vi "5492_AutonomousTurn.vi"(8 "error in (no error)":errorcluster, 10 "Yaw Goallll":dbl) -> (0 "error out (no error)":errorcluster)   [LabVIEW 2017]
uses:
  Public/Documents/Cross The Road Electronics/Phoenix-LabVIEW/Motor Controller/Controls/CTRE_Phoenix_MotorControl_ControlMode.ctl
  <vilib>/Rock Robotics/WPI/Utilities/WPI_GetSetVariantRefNum.vi
  <vilib>/Rock Robotics/WPI/RobotDrive/WPI_RobotDriveSafetyCheck.vi
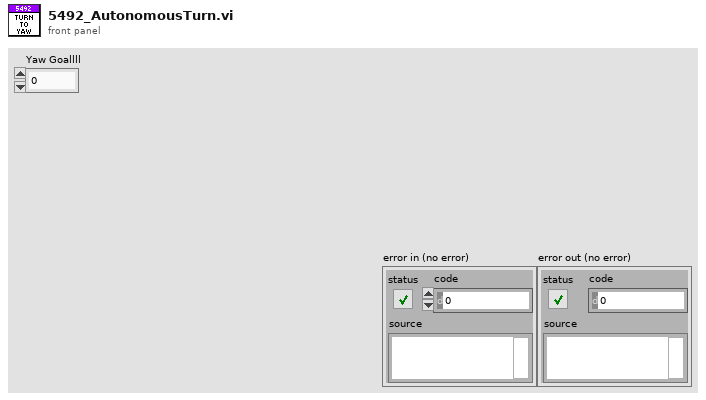
[diagram p1: front panel]
types:
  T1 = typedef "CTRE_Phoenix_MotorControl_ControlMode.ctl" = u16
  T2 = cluster{"Yaw":dbl, "Roll":dbl, "Pitch":dbl, "Heading":dbl, "Fused Heading":dbl}
  T3 = typedef "WPI_RobotDriveDevRef.ctl" = cluster{"DevStatus":errorcluster, "Motors[]":T4[], "Square Inputs":bool, "Max Output":dbl}
  T4 = typedef "WPI_MotorControlDeviceRef.ctl" = cluster{"DeviceStatus":errorcluster, "Type":T5, "PWM":cluster{"PWM Channel":T6, "DeadBand":T7}, "CAN":cluster{"Device Number":u8, "SetOutput VI Ref":variant, "GetOutput VI Ref":variant, "Enable VI Ref":variant, "Disable VI Ref":variant, "Data":variant}, "Invert":bool, "DIO PWM":cluster{"PWM \"Enable\" Channel":T6, "DIOChannel":T8, "PWM Rate":dbl}}
  T5 = typedef "WPI_MotorControlType.ctl" = enum16{"PWM", "CAN", "DIO PWM"}
  T6 = typedef "FPGA_DIOPWMChannel.ctl" = enum8{"PWM 0", "PWM 1", "PWM 2", "PWM 3", "PWM 4", "PWM 5", "PWM 6", "PWM 7", "PWM 8", "PWM 9", "PWM MXP 0", "PWM MXP 1", "PWM MXP 2", "PWM MXP 3", "PWM MXP 4", "PWM MXP 5", "PWM MXP 6", "PWM MXP 7", "PWM MXP 8", "PWM MXP 9", "Invalid"}
  T7 = typedef "WPI_PWMDeadband.ctl" = cluster{"Name":string, "maxPositivePwm":i32, "minPositivePwm":i32, "centerPwm":i32, "maxNegativePwm":i32, "minNegativePwm":i32, "angularRange":u16}
  T8 = typedef "FPGA_DIOChannel.ctl" = enum8{"DIO 0", "DIO 1", "DIO 2", "DIO 3", "DIO 4", "DIO 5", "DIO 6", "DIO 7", "DIO 8", "DIO 9", "DIO MXP 0", "DIO MXP 1", "DIO MXP 2", "DIO MXP 3", "DIO MXP 4", "DIO MXP 5", "DIO MXP 6", "DIO MXP 7", "DIO MXP 8", "DIO MXP 9", "DIO MXP 10", "DIO MXP 11", "DIO MXP 12", "DIO MXP 13", "DIO MXP 14", "DIO MXP 15", "SPI Port CS1", "SPI Port CS2", "SPI Port CS3", "SPI Port MISO", "SPI Port MOSI", "Invalid"}
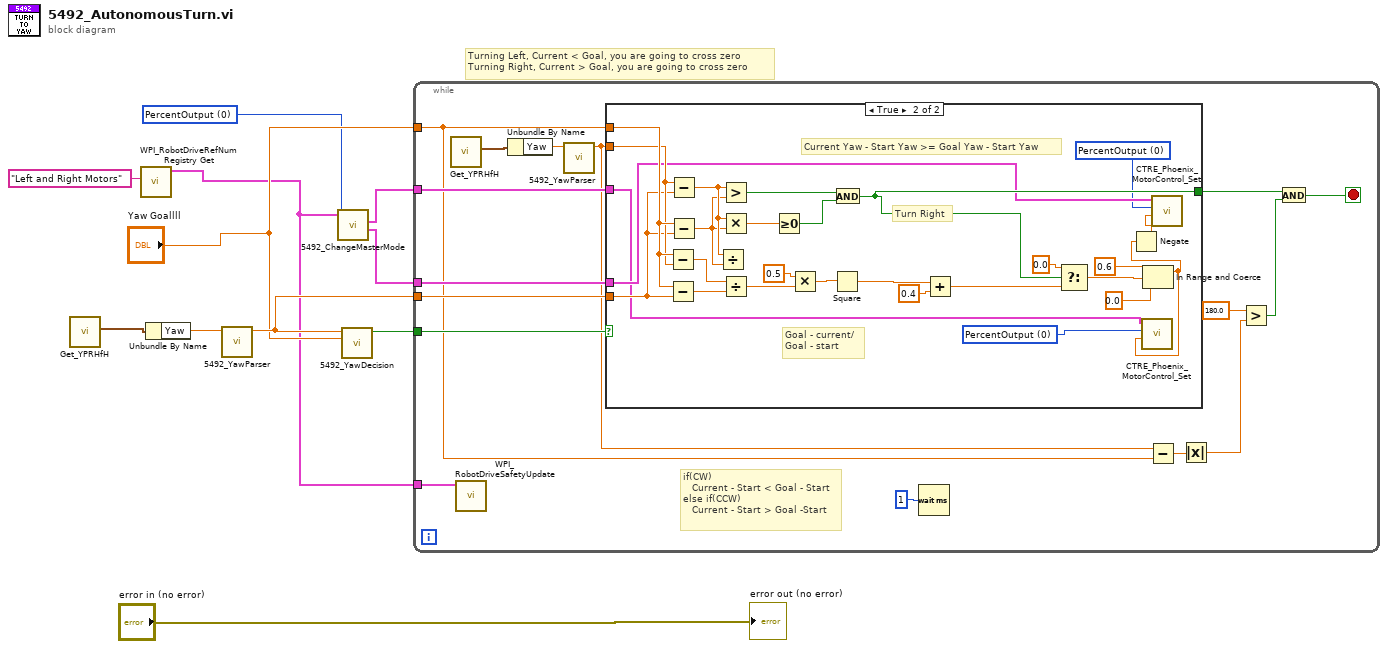
[diagram p0: block diagram]
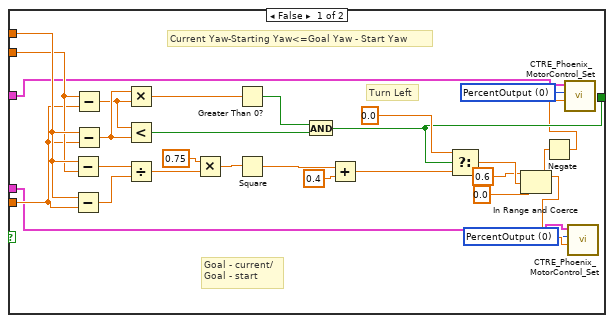
[diagram p2: hidden frame]
diagram:
  w3 = T1 0 items=["PercentOutput"=0, "Position"=1, "Velocity"=2, "Current"=3, "Follower"=5, "MotionProfile"=6, "MotionMagic"=7, "MotionMagicArc"=8, "MotionProfileArc"=10, "Disabled"=15] ("Control Mode")
  # "Turning Left, Current < Goal, you are going to cross zero\nTurning Right, Current > Goal, you are going to cross zero"
  n1 = call <vilib>:"Get_YPRHfH.vi"() -> ("YRPHfH"=w5:T2)  [unwired: 11 in]
  n2 = call <vilib>:"WPI_RobotDriveRefNum Registry Get.vi"("refnum name"="Left and Right Motors") -> ("RobotDriveDevRef"=w1:T3)  [unwired: 9 in, 1 out]
  n3 = Unbundle By Name(w5) -> ("Yaw"=w9:dbl)
  n4 = call "5492_YawParser.vi"("Yaw"=w9) -> ("Parsed Yaw"=w7:dbl)  [unwired: 10 in]
  n5 = call "5492_ChangeMasterMode.vi"("Control Mode"=w3, "RobotDriveDevRef"=w1) -> ("CAN Talon SRX Right"=w10:T4, "CAN Talon SRX Ref Left"=w11:T4)  [unwired: 7 in, 1 out]
  n6 = call "5492_YawDecision.vi"("Yaw Goallll"="Yaw Goallll", "Parsed Yaw"=w7) -> ("Right???"=w8:bool)  [unwired: 9 in]
  n7 = while {
    tunnel: w11 -> [w26]
    tunnel: w10 -> [w25]
    tunnel: w8 -> [w24]
    tunnel: w7 -> [w22]
    tunnel: "Yaw Goallll" -> [w19]
    tunnel: w1 -> [w12]
    stop <- w13 stop-if-true
    # "if(CW)\n   Current - Start < Goal - Start\nelse if(CCW)\n   Current - Start > Goal -Start"
    n8 = call <vilib>:"Get_YPRHfH.vi"() -> ("YRPHfH"=w21:T2)  [unwired: 11 in]
    n9 = call <vilib>:"WPI_RobotDriveSafetyUpdate.vi"("RobotDriveDevRef"=w12) -> ()  [unwired: 1 in, 10 out]
    n10 = Unbundle By Name(w21) -> ("Yaw"=w23:dbl)
    n11 = call "5492_YawParser.vi"("Yaw"=w23) -> ("Parsed Yaw"=w20:dbl)  [unwired: 10 in]
    n12 = case shown="True" w24 {
      tunnel: w26 -> [w33 w55]
      tunnel: w25 -> [w30 w60]
      tunnel: w20 -> [w39 w67]
      tunnel: w22 -> [w38 w66]
      tunnel: w19 -> [w40 w74]
      tunnel: [w53 w79] -> w14
      frame False {
        w28 = T1 0 items=["PercentOutput"=0, "Position"=1, "Velocity"=2, "Current"=3, "Follower"=5, "MotionProfile"=6, "MotionMagic"=7, "MotionMagicArc"=8, "MotionProfileArc"=10, "Disabled"=15] ("Control Mode")
        w31 = T1 0 items=["PercentOutput"=0, "Position"=1, "Velocity"=2, "Current"=3, "Follower"=5, "MotionProfile"=6, "MotionMagic"=7, "MotionMagicArc"=8, "MotionProfileArc"=10, "Disabled"=15] ("Control Mode")
        # "Current Yaw-Starting Yaw<=Goal Yaw - Start Yaw"
        # "Goal - current/\nGoal - start"
        # "Turn Left"
        n13 = Subtract(x=w40, y=w39) -> (x-y=w41:dbl)
        n14 = Subtract(x=w40, y=w38) -> (x-y=w42:dbl)
        n15 = Subtract(x=w39, y=w38) -> (x-y=w50:dbl)
        n16 = Subtract(x=w40, y=w38) -> (x-y=w51:dbl)
        n17 = Multiply(x=w51, y=w50) -> (x*y=w49:dbl)
        n18 = Less?(x=w50, y=w51) -> (x < y?=w52:bool)
        n19 = Divide(x=w41, y=w42) -> (x/y=w45:dbl)
        n20 = Multiply(x=0.75, y=w45) -> (x*y=w44:dbl)
        n21 = Greater Than 0?(x=w49) -> (x > 0?=w48:bool)
        n22 = Square(x=w44) -> (x^2=w43:dbl)
        n23 = And(x=w48, y=w52) -> (x .and. y?=w53:bool)
        n24 = Add(x=w43, y=0.4) -> (x+y=w37:dbl)
        n25 = Select(t=0.0, s=w53, f=w37) -> (s? t:f=w36:dbl)
        n26 = In Range and Coerce(upper limit=0.6, x=w36, lower limit=0.0) -> (coerced(x)=w29:dbl)  [unwired: 1 out]
        n27 = Negate(x=w29) -> (-x=w32:dbl)
        n28 = call "CTRE_Phoenix_MotorControl_Set.vi"("Output"=w32, "Control Mode"=w31, "PhoenixMotorControlDevRef"=w33) -> ()  [unwired: 7 in, 2 out]
        n29 = call "CTRE_Phoenix_MotorControl_Set.vi"("Output"=w29, "Control Mode"=w28, "PhoenixMotorControlDevRef"=w30) -> ()  [unwired: 7 in, 2 out]
      }
      frame True {
        w57 = T1 0 items=["PercentOutput"=0, "Position"=1, "Velocity"=2, "Current"=3, "Follower"=5, "MotionProfile"=6, "MotionMagic"=7, "MotionMagicArc"=8, "MotionProfileArc"=10, "Disabled"=15] ("Control Mode")
        w58 = T1 0 items=["PercentOutput"=0, "Position"=1, "Velocity"=2, "Current"=3, "Follower"=5, "MotionProfile"=6, "MotionMagic"=7, "MotionMagicArc"=8, "MotionProfileArc"=10, "Disabled"=15] ("Control Mode")
        # "Current Yaw - Start Yaw >= Goal Yaw - Start Yaw"
        # "Goal - current/\nGoal - start"
        # "Turn Right"
        n30 = Subtract(x=w74, y=w67) -> (x-y=w73:dbl)
        n31 = Subtract(x=w74, y=w66) -> (x-y=w72:dbl)
        n32 = Subtract(x=w67, y=w66) -> (x-y=w76:dbl)
        n33 = Subtract(x=w74, y=w66) -> (x-y=w75:dbl)
        n34 = Divide(x=w76, y=w75) -> ()  [unwired: 1 out]
        n35 = Greater?(x=w76, y=w75) -> (0:w80:bool)
        n36 = Multiply(x=w76, y=w75) -> (x*y=w78:dbl)
        n37 = Divide(x=w73, y=w72) -> (x/y=w69:dbl)
        n38 = Greater Or Equal To 0?(x=w78) -> (x >= 0?=w77:bool)
        n39 = Multiply(x=0.5, y=w69) -> (x*y=w70:dbl)
        n40 = Square(x=w70) -> (x^2=w71:dbl)
        n41 = And(x=w80, y=w77) -> (x .and. y?=w79:bool)
        n42 = Add(x=w71, y=0.4) -> (x+y=w64:dbl)
        n43 = Select(t=0.0, s=w79, f=w64) -> (s? t:f=w62:dbl)
        n44 = In Range and Coerce(upper limit=0.6, x=w62, lower limit=0.0) -> (coerced(x)=w56:dbl)  [unwired: 1 out]
        n45 = Negate(x=w56) -> (-x=w59:dbl)
        n46 = call "CTRE_Phoenix_MotorControl_Set.vi"("Output"=w56, "Control Mode"=w57, "PhoenixMotorControlDevRef"=w55) -> ()  [unwired: 7 in, 2 out]
        n47 = call "CTRE_Phoenix_MotorControl_Set.vi"("Output"=w59, "Control Mode"=w58, "PhoenixMotorControlDevRef"=w60) -> ()  [unwired: 7 in, 2 out]
      }
    }
    n48 = Wait (ms)(milliseconds to wait=u32 1) -> ()  [unwired: 1 out]
    n49 = Subtract(x=w20, y=w19) -> (x-y=w18:dbl)
    n50 = Absolute Value(x=w18) -> (abs(x)=w17:dbl)
    n51 = Greater?(x=180.0, y=w17) -> (0:w15:bool)
    n52 = And(x=w14, y=w15) -> (x .and. y?=w13:bool)
  }
  "error out (no error)" <- "error in (no error)"
